vi "认识for循环.vi"() -> ()   [LabVIEW 2018]
panel:
  out "数字(0-1)":dbl
  out "数组 2":dbl[](array[numeric])
  out "外循环i":i32
  out "内循环i":i32
  out "数组":dbl[][](array[numeric])
  in  "循环次数":i32
  in  "停止":bool
  out "字符串":string="FOR循环是一种先检查条件后执行的循环方式\n主要用于判定循环的次数"
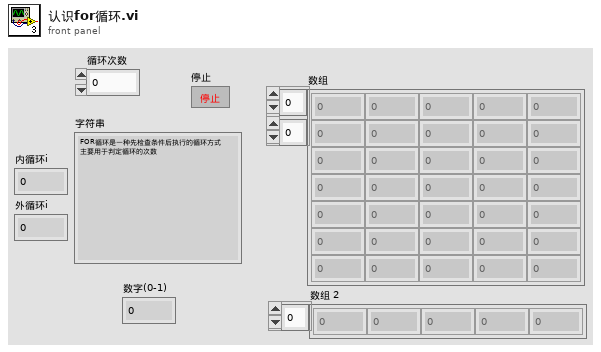
[diagram p1: front panel]
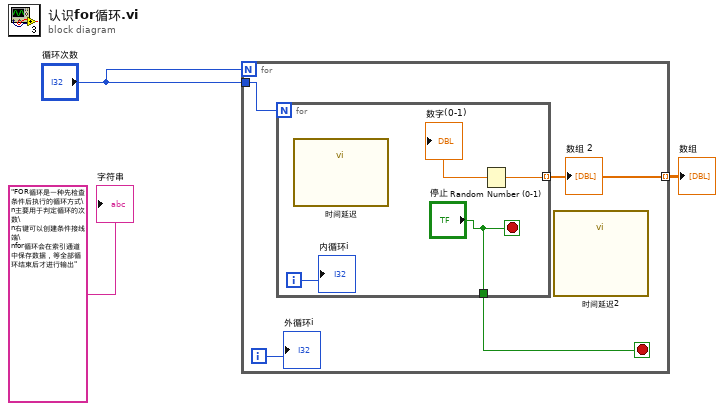
[diagram p0: block diagram]
diagram:
  n1 = for {
    N: "循环次数" -> [_]
    tunnel: [w7] -> w1 mode=indexing
    tunnel: "循环次数" -> [w6]
    i -> [w4]
    stop <- w5 stop-if-true
    n2 = for {
      N: w6 -> [_]
      tunnel: [w10] -> w7 mode=indexing
      tunnel: ["停止"] -> w5
      i -> [w8]
      stop <- "停止" stop-if-true
      n3 = call "时间延迟"() -> ()  [unwired: 11 in, 1 out]
      n4 = Random Number (0-1)() -> (number: 0 to 1=w10:dbl)
      "数字(0-1)" <- w10
      "内循环i" <- w8
    }
    "数组 2" <- w7
    n5 = call "时间延迟2"() -> ()  [unwired: 11 in, 1 out]
    "外循环i" <- w4
  }
  "数组" <- w1
  "字符串" <- "FOR循环是一种先检查条件后执行的循环方式\n主要用于判定循环的次数\n右键可以创建条件接线端\nfor循环会在索引通道中保存数据，等全部循环结束后才进行输出"
